vi "Handle Message.vi"(8 "error in (no error)":errorcluster, 9 "Message Completion Handler":refnum<class "Message Completion Handler.lvclass">, 10 "Message":string, 11 "RandomNumberGenerator in":refnum<class "RandomNumberGenerator.lvclass">) -> (0 "error out":errorcluster, 1 "Synchronously Complete Message?":bool=TRUE, 2 "Message Response":string, 3 "RandomNumberGenerator out":refnum<class "RandomNumberGenerator.lvclass">)   [LabVIEW 2020, in "RandomNumberGenerator.lvlib" / "RandomNumberGenerator.lvclass"]
doc: "<b>Handle Message</b>\nThis method allows you to handle messages received from other plugins/services. If you don't put handlers here for messages, then all messages broadcast to plugins will be thrown away by this plugin. If you need to handle a specific message (like pause, resume, etc.) the handler needs to be written here."
uses:
  RandomNumberGenerator.lvclass
  RandomNumberGenerator.lvclass/RandomNumberGenerator.ctl
  <vilib>/ADAS Record/Utilities/TypeDefs/ADAS gRPC/DataStreamGrpc Message.ctl
  <vilib>/ADAS Record/Utilities/ADAS Utilities.lvlib
  <vilib>/FlexLogger/SDK/PluginSDK.lvlibp/PEFClasses/SDK/Message Completion Handler/Message Completion Handler.lvclass
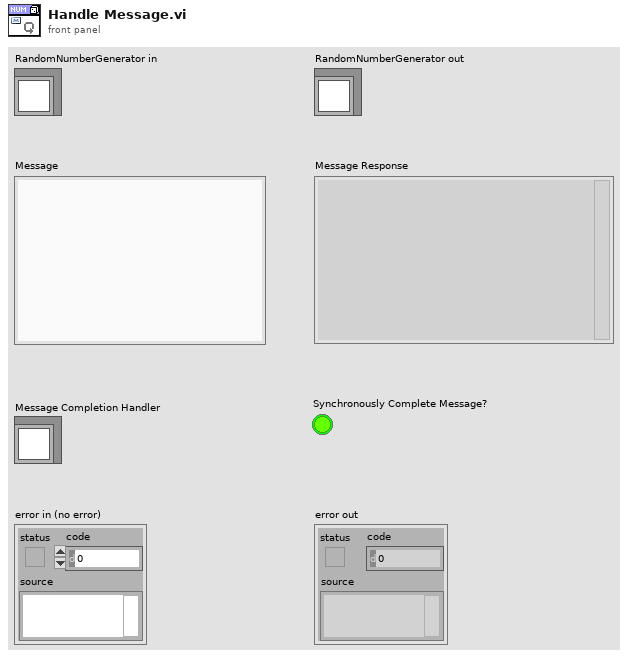
[diagram p1: front panel]
types:
  T1 = typedef "ADAS Utilities.lvlib/DataStreamGrpc Message.ctl" = cluster{"messageName":string, "details":string}
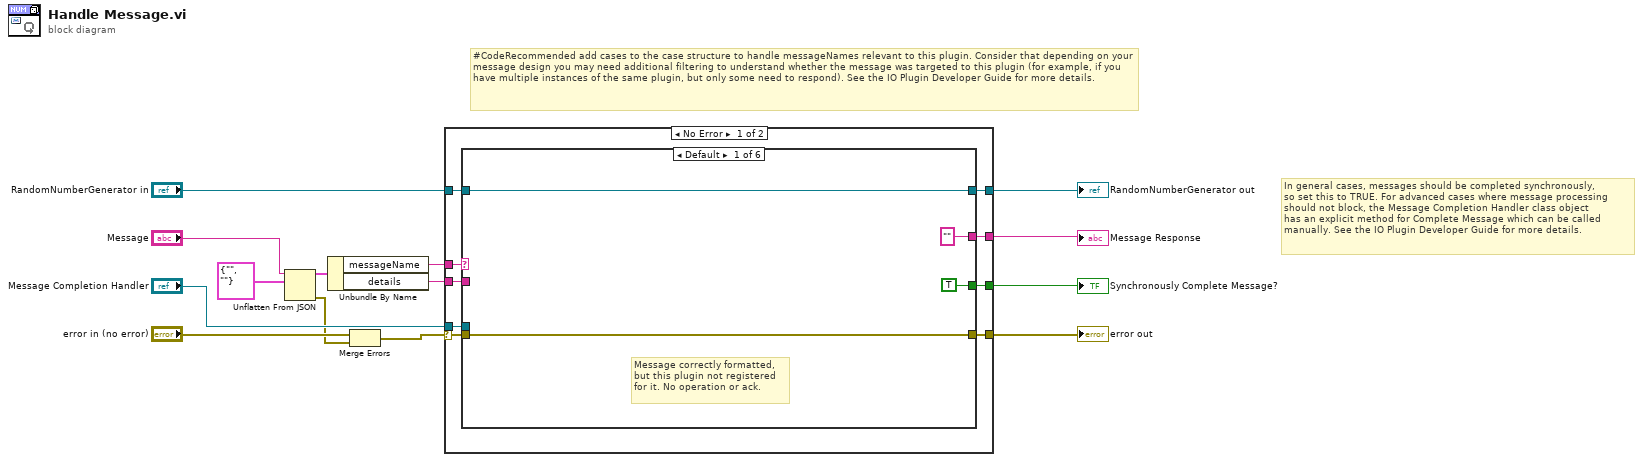
[diagram p0: block diagram]
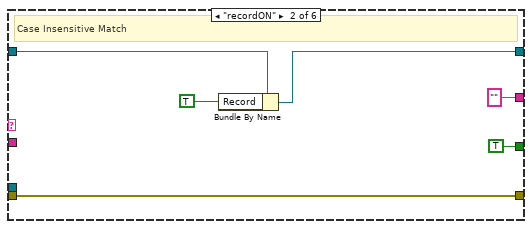
[diagram p2: hidden frame]
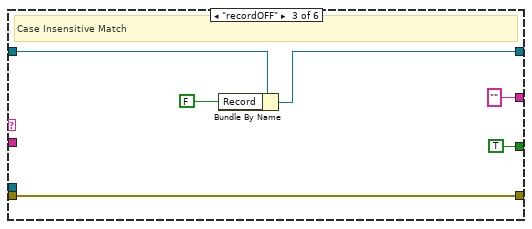
[diagram p3: hidden frame]
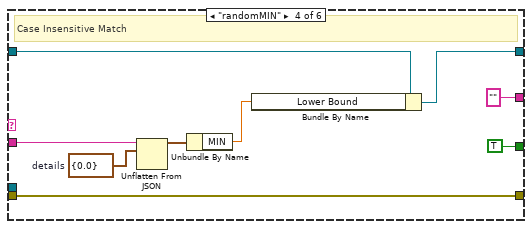
[diagram p4: hidden frame]
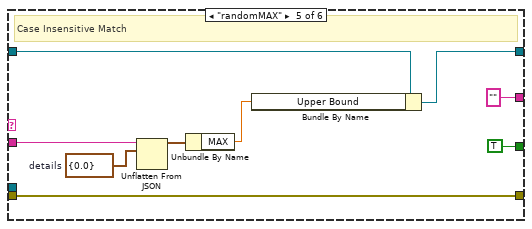
[diagram p5: hidden frame]
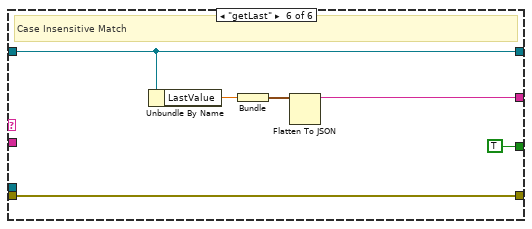
[diagram p6: hidden frame]
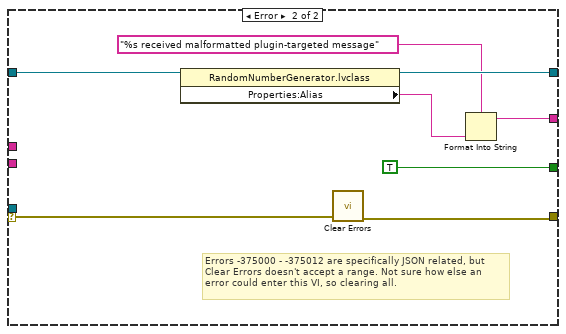
[diagram p7: hidden frame]
diagram:
  # "In general cases, messages should be completed synchronously,\nso set this to TRUE. For advanced cases where message processing\nshould not block, the Message Completion Handler class object\nhas an explicit method for Complete Message which can be called\nmanually. See the IO Plugin Developer Guide for more details."
  # "#CodeRecommended add cases to the case structure to handle messageNames relevant to this plugin. Consider that depending on your message design you may need additional filtering to understand whether the message was targeted to this plugin (for example, if you have multiple instances of the same plugin, but only some need to respond). See the IO Plugin Developer Guide for more details."
  n1 = Unflatten From JSON(JSON string="Message", type and defaults=T1 {"messageName"="", "details"=""} ("DataStreamGrpc Message")) -> (value=w7:T1, error out=w1:errorcluster)  [unwired: 5 in]
  n2 = Unbundle By Name(w7) -> ("messageName"=w6:string, "details"=w5:string)
  n3 = Merge Errors("error in (no error)", w1) -> (w2:errorcluster)
  n4 = case shown="No Error" w2 {
    selector: w2 -> [w15 w71]
    tunnel: [w23 w70] -> w14
    tunnel: [w22 w67] -> w13
    tunnel: "Message Completion Handler" -> [w21 _]
    tunnel: "RandomNumberGenerator in" -> [w20 w68]
    tunnel: w6 -> [w19 _]
    tunnel: w5 -> [w18 _]
    tunnel: [w17 w64] -> w4
    tunnel: [w16 TRUE ("Synchronously Complete Message?")] -> w3
    frame No Error {
      n5 = case shown="Default" w19 {
        tunnel: [w27 w33 w39 w48 w57 w63] -> w23
        tunnel: [w26 w29 w35 w44 w53 w61] -> w22
        tunnel: w15 -> [w27 w33 w39 w48 w57 w63]
        tunnel: w21 -> [_ _ _ _ _ _]
        tunnel: w20 -> [w26 w30 w36 w45 w54 w61]
        tunnel: w18 -> [_ _ _ w43 w52 _]
        tunnel: ["" ("Message Response") "" ("Message Response") "" ("Message Response") "" ("Message Response") "" ("Message Response") w58] -> w17
        tunnel: [TRUE ("Synchronously Complete Message?") TRUE ("Synchronously Complete Message?") TRUE ("Synchronously Complete Message?") TRUE ("Synchronously Complete Message?") TRUE ("Synchronously Complete Message?") TRUE ("Synchronously Complete Message?")] -> w16
        frame Default {
          # "Message correctly formatted,\nbut this plugin not registered\nfor it. No operation or ack."
        }
        frame "recordON" {
          # "Case Insensitive Match"
          n6 = Bundle By Name(cluster=w30, "Record"=TRUE) -> (w29:refnum<class "RandomNumberGenerator.lvclass">)
        }
        frame "recordOFF" {
          # "Case Insensitive Match"
          n7 = Bundle By Name(cluster=w36, "Record"=FALSE) -> (w35:refnum<class "RandomNumberGenerator.lvclass">)
        }
        frame "randomMIN" {
          w42 = cluster{"MIN":dbl} {"MIN"=0.0}  # details
          # "Case Insensitive Match"
          n8 = Unflatten From JSON(JSON string=w43, type and defaults=w42) -> (value=w41:cluster{"MIN":dbl})  [unwired: 5 in, 1 out]
          n9 = Unbundle By Name(w41) -> ("MIN"=w40:dbl)
          n10 = Bundle By Name(cluster=w45, "Lower Bound"=w40) -> (w44:refnum<class "RandomNumberGenerator.lvclass">)
        }
        frame "randomMAX" {
          w51 = cluster{"MAX":dbl} {"MAX"=0.0}  # details
          # "Case Insensitive Match"
          n11 = Unflatten From JSON(JSON string=w52, type and defaults=w51) -> (value=w50:cluster{"MAX":dbl})  [unwired: 5 in, 1 out]
          n12 = Unbundle By Name(w50) -> ("MAX"=w49:dbl)
          n13 = Bundle By Name(cluster=w54, "Upper Bound"=w49) -> (w53:refnum<class "RandomNumberGenerator.lvclass">)
        }
        frame "getLast" {
          # "Case Insensitive Match"
          n14 = Unbundle By Name(w61) -> ("LastValue"=w60:dbl)
          n15 = Bundle("LastValue"=w60) -> (w59:cluster{"LastValue":dbl})  [unwired: 1 in]
          n16 = Flatten To JSON(anything=w59) -> (JSON string=w58:string)  [unwired: 2 in, 1 out]
        }
      }
    }
    frame Error {
      # "Errors -375000 - -375012 are specifically JSON related, but \nClear Errors doesn't accept a range. Not sure how else an \nerror could enter this VI, so clearing all."
      n17 = property class="RandomNumberGenerator.lvclass"(reference=w68) -> (reference out=w67:refnum<class "RandomNumberGenerator.lvclass">, "Properties:Alias"=w65:string)  [unwired: 1 in, 1 out]
      n18 = call <vilib>:"Clear Errors.vi"("error in (no error)"=w71) -> ("error out"=w70:errorcluster)  [unwired: 5 in, 1 out]
      n19 = Format Into String(format string="%s received malformatted plugin-targeted message", w65) -> (resulting string=w64:string)  [unwired: 2 in, 1 out]
    }
  }
  "error out" <- w14
  "RandomNumberGenerator out" <- w13
  "Message Response" <- w4
  "Synchronously Complete Message?" <- w3
